vi "BRig_Host__Loop_Consumer_RunState__BlockData.vi"(4 "threshold_2":u16, 6 "threshold_1":u16, 9 "input_idx":i32[](array[numeric]), 10 "input_dataTS":u16[][](array[numeric]), 11 "input_dataPlot":u16[][](array[numeric])) -> (0 "output_newData":bool, 1 "output_idx":i32[](array[numeric]), 2 "output_dataTS":u16[][](array[numeric]), 3 "output_dataPlot":u16[][](array[numeric]))   [LabVIEW 2014]
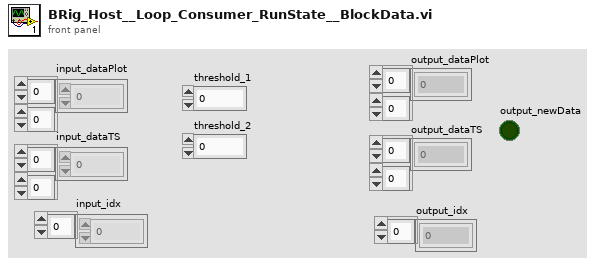
[diagram p1: front panel]
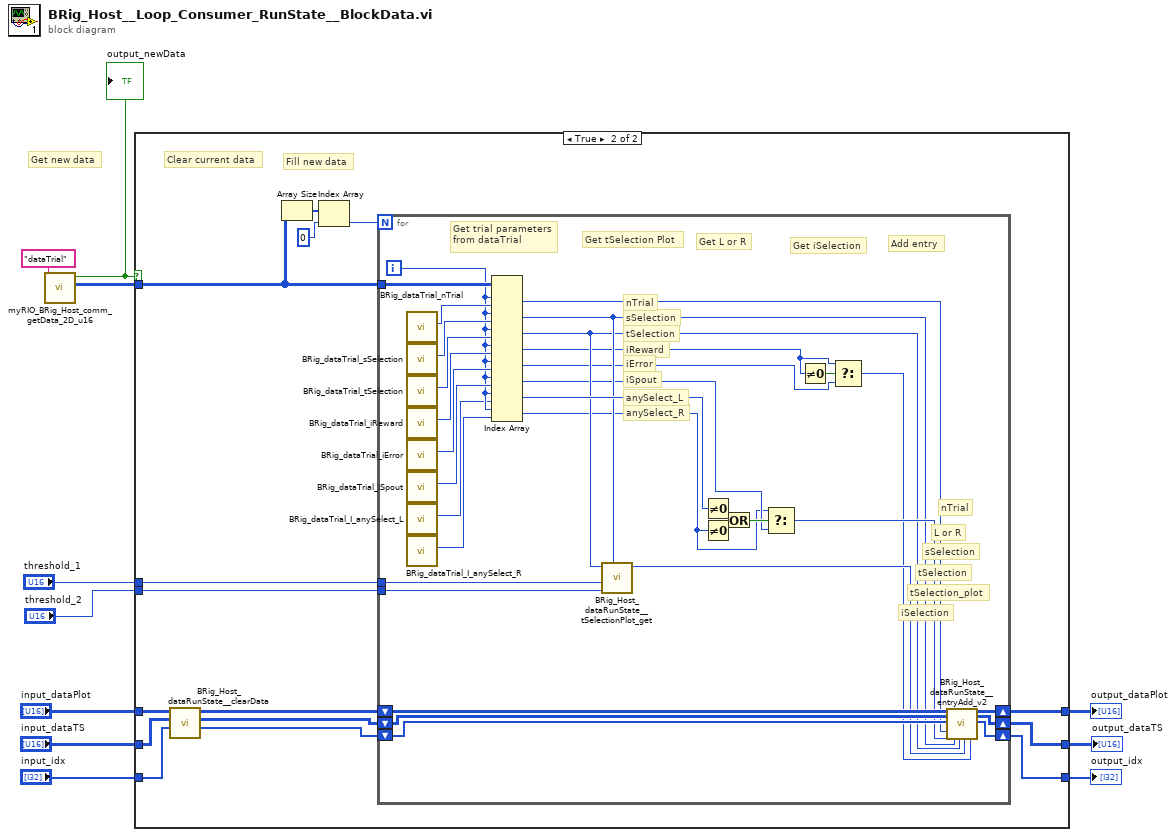
[diagram p0: block diagram]
diagram:
  # "Get new data"
  n1 = call "myRIO_BRig_Host_comm_getData_2D_u16.vi"("input_fileName"="dataTrial") -> ("output_data_2D"=w9:u16[][], "output_I_data"=w10:bool)  [unwired: 9 in]
  "output_newData" <- w10
  n2 = case shown="True" w10 {
    tunnel: w9 -> [_ w27]
    tunnel: "input_dataPlot" -> [w14 w26]
    tunnel: "input_dataTS" -> [w13 w25]
    tunnel: "input_idx" -> [w12 w24]
    tunnel: [w14 w18] -> w5
    tunnel: [w13 w17] -> w4
    tunnel: [w12 w16] -> w3
    tunnel: "threshold_1" -> [_ w23]
    tunnel: "threshold_2" -> [_ w22]
    frame False {
    }
    frame True {
      # "Fill new data"
      # "Clear current data"
      n3 = call "BRig_Host_dataRunState__clearData.vi"("input_idx"=w24, "input_dataTS"=w25, "input_dataPlot"=w26) -> ("output_idx"=w19:i32[], "output_dataTS"=w20:u16[][], "output_dataPlot"=w21:u16[][])  [unwired: 6 in]
      n4 = Array Size(array=w27) -> (size(s)=w29:i32[])
      n5 = Index Array(array=w29, index=0) -> (element=w15:i32)
      n6 = for {
        N: w15 -> [_]
        tunnel: w27 -> [w62]
        tunnel: w23 -> [w52]
        tunnel: w22 -> [w51]
        shift-right: [w47] -> w18
        shift-left: w21 -> [w50]
        shift-right: [w46] -> w17
        shift-left: w20 -> [w49]
        shift-right: [w45] -> w16
        shift-left: w19 -> [w48]
        i -> [w55]
        # "iSelection"
        # "tSelection_plot"
        # "nTrial"
        # "sSelection"
        # "tSelection"
        # "L or R"
        # "nTrial"
        # "sSelection"
        # "tSelection"
        # "iReward"
        # "iError"
        # "iSpout"
        # "anySelect_L"
        # "anySelect_R"
        # "Get iSelection"
        # "Get L or R"
        # "Add entry"
        # "Get tSelection Plot"
        # "Get trial parameters\nfrom dataTrial"
        n7 = call "BRig_dataTrial_nTrial.vi"() -> ("output_nTrial"=w61:i32)  [unwired: 11 in]
        n8 = call "BRig_dataTrial_sSelection.vi"() -> ("output_sSelection"=w60:i32)  [unwired: 11 in]
        n9 = call "BRig_dataTrial_tSelection.vi"() -> ("output_tSelection"=w59:i32)  [unwired: 11 in]
        n10 = call "BRig_dataTrial_iReward.vi"() -> ("output_iReward"=w58:i32)  [unwired: 11 in]
        n11 = call "BRig_dataTrial_iError.vi"() -> ("output_iError"=w57:i32)  [unwired: 11 in]
        n12 = call "BRig_dataTrial_iSpout.vi"() -> ("output_iSpout"=w56:i32)  [unwired: 11 in]
        n13 = call "BRig_dataTrial_I_anySelect_L.vi"() -> ("output_I_allReward_L"=w54:i32)  [unwired: 11 in]
        n14 = call "BRig_dataTrial_I_anySelect_R.vi"() -> ("output_I_anySelect_R"=w53:i32)  [unwired: 11 in]
        n15 = Index Array(array=w62, index (row) #1=w55, index (col) #1=w61, index (row) #2=w55, index (col) #2=w60, index (row) #3=w55, index (col) #3=w59, index (row) #4=w55, index (col) #4=w58, index (row) #5=w55, index (col) #5=w57, index (row) #6=w55, index (col) #6=w56, index (row) #7=w55, index (col) #7=w54, index (row) #8=w55, index (col) #8=w53) -> (element #1=w44:u16, element #2=w38:u16, element #3=w37:u16, element #4=w34:u16, element #5=w33:u16, element #6=w31:u16, element #7=w40:u16, element #8=w30:u16)
        n16 = call "BRig_Host_dataRunState__tSelectionPlot_get.vi"("input_sSelection"=w38, "input_threshold_2"=w51, "input_threshold_1"=w52, "input_tSelection"=w37) -> ("output_tSelection_plot"=w36:u16)  [unwired: 7 in]
        n17 = Not Equal To 0?(x=w40) -> (x != 0?=w42:bool)
        n18 = Not Equal To 0?(x=w30) -> (x != 0?=w43:bool)
        n19 = Or(x=w42, y=w43) -> (x .or. y?=w41:bool)
        n20 = Select(t=w30, s=w41, f=w31) -> (s? t:f=w39:u16)
        n21 = Not Equal To 0?(x=w34) -> (x != 0?=w35:bool)
        n22 = Select(t=w34, s=w35, f=w33) -> (s? t:f=w32:u16)
        n23 = call "BRig_Host_dataRunState__entryAdd_v2.vi"("input_dataPlot"=w50, "input_dataTS"=w49, "input_idx"=w48, "input_nTrial"=w44, "input_LorR"=w39, "input_sSelection"=w38, "input_tSelection"=w37, "input_tSelectionPlot"=w36, "input_iSelection"=w32) -> ("output_dataPlot"=w47:u16[][], "output_dataTS"=w46:u16[][], "output_idx"=w45:i32[])  [unwired: 7 in, 1 out]
      }
    }
  }
  "output_dataPlot" <- w5
  "output_dataTS" <- w4
  "output_idx" <- w3
